vi "MAIN only-save-v3.vi"(0 "VISA resource name":refnum<visa-resource-name>="COM1", 1 "baud rate":u32=9600, 3 "bytes to read":u32=1000, 4 "data bits":u16=8 min=5 max=8 step=1, 5 "parity":u16(ring) items=["None", "Odd", "Even", "Mark", "Space"], 7 "stop bits":u16(ring)=10 items=["1.0"=10, "1.5"=15, "2.0"=20], 9 "XON Character":u8=17 format="%.0x", 13 "string to write":string="*IDN?", 14 "XOFF Character":u8=19 format="%.0x", 15 "timeout (ms)":u32=10000, 17 "write":bool=TRUE, 21 "End read on termination character?":bool=TRUE, 24 "termination char\n(0xA = '\\n' = LF)":u8=10 format="%.0x", 25 "Input\nbuffer size":u32=4096, 26 "read":bool=TRUE) -> (20 "read string":string)   [LabVIEW 2012]
doc: "The Advanced Serial Read and Write example performs a Serial Port Read, a Serial Port Write, or a combination of these actions while setting some advanced serial features like buffer size, termination characters, and XON/XOFF flow control. The user selects the actions (read or write) on the front panel. If both are selected, the VI will write the data first, read the data and then close the VISA session that is opened to the port. \n\nThe parameters set for the serial port must match the parameters of the connected instrument or device. In this example, the bytes to read parameter specifies the number of bytes that the serial port reads. If there were more bytes at the port than the number specified in bytes to read, those bytes would not be read. Also, if you specify to read more bytes than the number of bytes actually read, you might receive a timeout error message.\n\nINSTRUCTIONS:\n1) Select the serial resource and configuration parameters (baud rate, data bits, parity, stop bits, flow control).\n2) Termination character can be enabled and set. Also, set the required input buffer size prior to running the example.\n3) Select the operations to be performed. \n4) Connect the serial port to your device. If no device is available, perform a loopback test by doing one of the following. Short pins 2 and 3 on a RS-232 cable or short pin 4 to pin 8 and pin 5 to pin 9 on a RS-485/422 cable. \n5) Run the VI to see the data read. (The \"read string\" will match the \"string to write\" if a loopback test was performed.)\n\nThis example exposes several advanced features that you may need for your application. Not all applications need all the features shown in this example. The input buffer size is likely an important setting that you want to control in your application. This example expands upon the flow control option for XON and XOFF, allowing the user to choose those control characters. The timeout parameter has been brought to the front panel so a user can specify the time period the VISA Read will wait for the number of bytes to read before timing out. Also, the user has several controls for the termination character, which is discussed later.\n\nNote that you can press the write and read buttons and change the bytes to read parameters on the fly, while the example is running. However, you must stop the example to change the other configuration parameters after the example has started running, and then run again.\n\nSet the I/O buffer size slightly higher the amount of data you expect to receive. This is very important for applications that don't use flow control, as you may lose characters if the receive buffer overflows.\n\nSetting the timeout period ensures that the operation returns with a timeout error if the operation cannot be performed in the specified time period. \n\nSome devices require a termination character in order to identify the end of command strings. Some devices send a termination character to signify the end of data to be read. \n\nThis example shows how you can end the Read operation once a termination character is detected in the buffer and/or append a termination character at the end of the Write data. To enable the Read to end on a termination character, use the VISA Configure Serial Port or use the VISA Properties Serial End Mode for Reads, Termination Character Enable, and Termination Character. To end the Write with a termination character, use the VISA Properties Serial End Mode for Writes, the Send End Enable, and Termination Character. In this example, the same termination character is used for both the Read and the Write. You can specify two different characters for your application, if desired.\n\nYour application may require specific characters for the XON/XOFF Flow Control. You can specify these characters with the VISA Properties Flow Control XOFF Character and Flow Control XON Character. Note that if the standard XON and XOFF characters are used, then decimal 17 and 19 are unavailable for data values. Remember that using flow control and setting an adequate buffer size allow you to prevent buffer overflows."
uses:
  <vilib>/Instr/_visa.llb/VISA Configure Serial Port (Instr).vi
panel:
  out "actual bytes read":u32
  in  "stop":bool
  in  "flow control":u16(ring) items=["None"=0, "XON/XOFF"=1, "RTS/CTS"=2, "DTR/DSR"=4]
  in  "End write with termination character?":bool=TRUE
  # "On Windows/Linux, consider using the Instrument Driver Finder (Help>>Find Instrument Drivers) to search for an instrument driver for your instrument."
  # "Select the serial resource and the operations to be performed.  If all are selected, the VI will write the data first, read data and then close the VISA session that is opened to the port.  This VI will wait until the specified number of bytes is received at the port, until the timeout period is met, or until a termination character is received.  The default termination character in this example is the Line Feed ( ASCII 0xA, '\\n' ).  Also, set the required input buffer size prior to running the example.\nNote: The example loops until the STOP button is pressed."
  # "For additional information select File >> VI Properties >> Documentation"
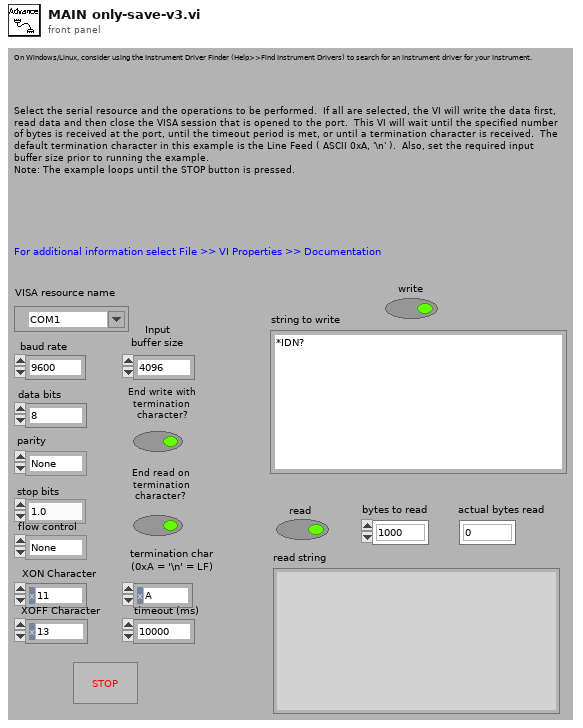
[diagram p1: front panel]
types:
  T1 = enum16{"open", "replace", "create", "open or create", "replace or create", "replace or create with confirmation"}
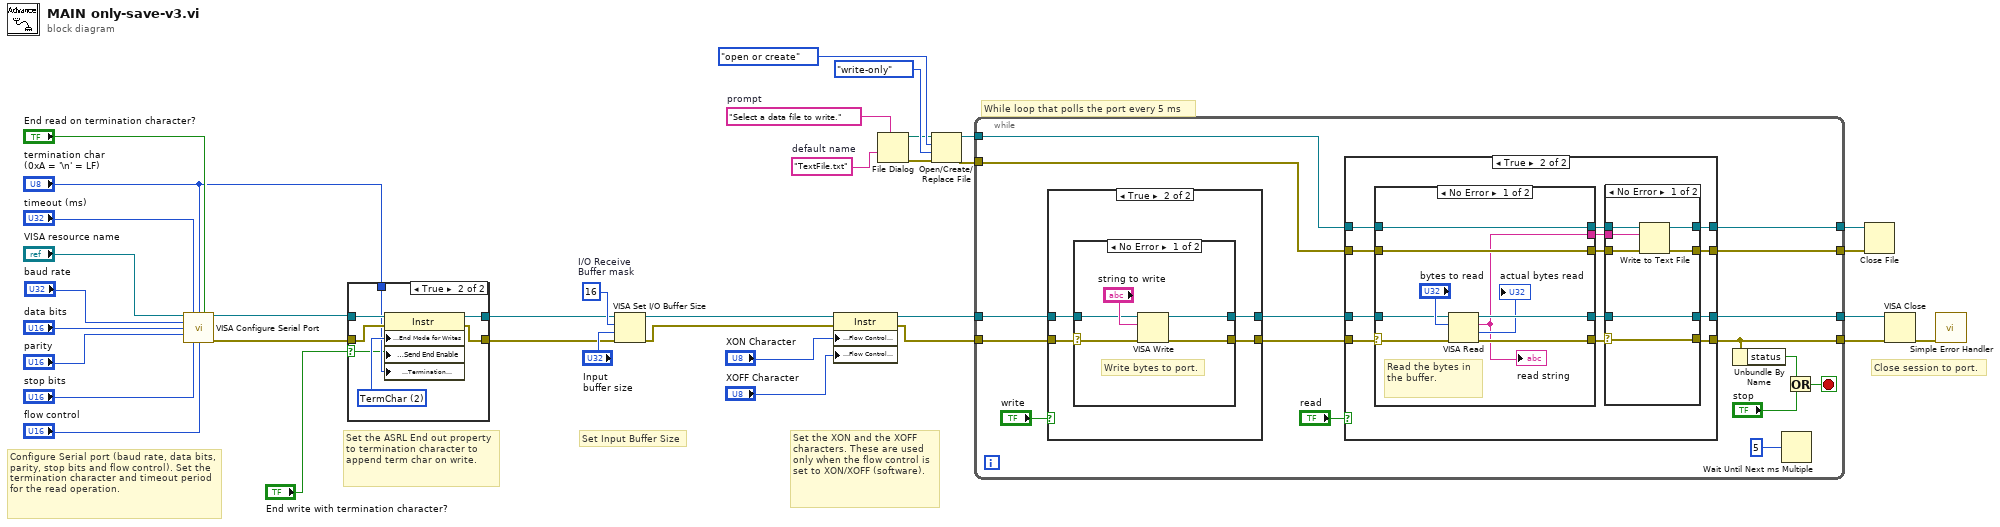
[diagram p0: block diagram]
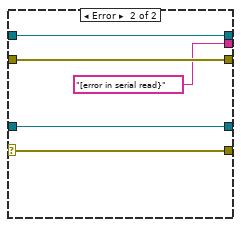
[diagram p7: hidden frame]
diagram:
  w6 = "TextFile.txt"  # default name
  w7 = "Select a data file to write."  # prompt
  w28 = u16 16  # I/O Receive Buffer mask
  # "While loop that polls the port every 5 ms"
  # "Set the XON and the XOFF characters. These are used only when the flow control is set to XON/XOFF (software)."
  # "Configure Serial port (baud rate, data bits, parity, stop bits and flow control). Set the termination character and timeout period for the read operation."
  # "Set Input Buffer Size"
  # "Set the ASRL End out property to termination character to append term char on write."
  # "Close session to port."
  n1 = call-poly "VISA Configure Serial Port"("VISA resource name"="VISA resource name", "timeout (10sec)"="timeout (ms)", "termination char\n(0xA = '\\n' = LF)"="termination char\n(0xA = '\\n' = LF)", "Enable Termination\nChar (T)"="End read on termination character?", "baud rate (9600)"="baud rate", "data bits (8)"="data bits", "parity (0:none)"="parity", "stop bits (10: 1 bit)"="stop bits", "flow control (0:none)"="flow control") -> ("VISA resource name out"=w14:refnum<visa-resource-name>, "error out"=w17:errorcluster)  [unwired: 1 in, 4 out]
  n2 = case shown="True" "End write with termination character?" {
    selector: "End write with termination character?" -> [_ w38]
    tunnel: w14 -> [w36 w44]
    tunnel: w17 -> [w37 w43]
    tunnel: [w36 w42] -> w15
    tunnel: [w37 w41] -> w16
    tunnel: "termination char\n(0xA = '\\n' = LF)" -> [_ w39]
    frame False {
    }
    frame True {
      w40 = u16 2 items=["None", "LastBit", "TermChar", "Break"] ("Serial Settings:Serial End Mode for Writes")
      n3 = property class="Instr"(reference=w44, error in=w43, "Serial Settings:End Mode for Writes"=w40, "Message Based Settings:Send End Enable"=w38, "Message Based Settings:Termination Character"=w39) -> (reference out=w42:refnum<visa-resource-name>, error out=w41:errorcluster)
    }
  }
  n4 = VISA Set I/O Buffer Size(VISA resource name=w15, mask (16)=w28, size (4096)="Input\nbuffer size", error in (no error)=w16) -> (VISA resource name out=w23:refnum<visa-resource-name>, error out=w22:errorcluster)
  n5 = property class="Instr"(reference=w23, error in=w22, "Serial Settings:Flow Control XON Character"="XON Character", "Serial Settings:Flow Control XOFF Character"="XOFF Character") -> (reference out=w13:refnum<visa-resource-name>, error out=w19:errorcluster)
  n6 = File Dialog(7:w7, 9:w6) -> (0:w8:errorcluster, 3:w5:path)  [unwired: 1 in, 6 out]
  n7 = Open/Create/Replace File(file path (use dialog)=w5, error in=w8, operation (0:open)=T1."open or create", access (0:read/write)=enum16{"read/write", "read-only", "write-only"}."write-only") -> (refnum out=w1:refnum<file>, error out=w2:errorcluster)  [unwired: 3 out]
  n8 = while {
    tunnel: w19 -> [w53]
    tunnel: w13 -> [w54]
    tunnel: [w52] -> w12
    tunnel: [w51] -> w11
    tunnel: [w48] -> w4
    tunnel: [w47] -> w3
    tunnel: w2 -> [w45]
    tunnel: w1 -> [w46]
    stop <- w50 stop-if-true
    n9 = case shown="True" "write" {
      tunnel: [w62 w66] -> w57
      tunnel: [w61 w65] -> w56
      tunnel: w54 -> [w62 w64]
      tunnel: w53 -> [w61 w63]
      frame False {
      }
      frame True {
        n10 = case shown="No Error" w63 {
          selector: w63 -> [w67 w73]
          tunnel: [w71 w72] -> w66
          tunnel: [w70 w73] -> w65
          tunnel: w64 -> [w68 w72]
          frame No Error {
            # "Write bytes to port."
            n11 = VISA Write(VISA resource name=w68, write buffer="string to write", error in (no error)=w67) -> (VISA resource name out=w71:refnum<visa-resource-name>, error out=w70:errorcluster)  [unwired: 1 out]
          }
          frame Error {
          }
        }
      }
    }
    n12 = case shown="True" "read" {
      tunnel: w56 -> [w76 w90]
      tunnel: w57 -> [w77 w89]
      tunnel: [w76 w79] -> w51
      tunnel: [w77 w81] -> w52
      tunnel: [w74 w83] -> w48
      tunnel: [w75 w85] -> w47
      tunnel: w46 -> [w75 w88]
      tunnel: w45 -> [w74 w87]
      frame False {
      }
      frame True {
        n13 = case "Read bytes from port." shown="No Error" w90 {
          selector: w90 -> [w106 w114]
          tunnel: [w109 w114] -> w80
          tunnel: [w110 w115] -> w82
          tunnel: w89 -> [w107 w115]
          tunnel: [w104 w112] -> w84
          tunnel: [w102 w113] -> w86
          tunnel: w88 -> [w102 w113]
          tunnel: w87 -> [w104 w112]
          tunnel: [w103 "[error in serial read}" ("read buffer")] -> w78
          frame No Error {
            # "Read the bytes in the buffer."
            n14 = VISA Read(VISA resource name=w107, byte count="bytes to read", error in (no error)=w106) -> (VISA resource name out=w110:refnum<visa-resource-name>, read buffer=w103:string, return count=→"actual bytes read":u32, error out=w109:errorcluster)
            "read string" <- w103
          }
          frame Error {
            # "Error occurred \nreading Bytes at \nSerial Port"
          }
        }
        n15 = case "Read bytes from port." shown="No Error" w80 {
          selector: w80 -> [w97 w98]
          tunnel: [w97 w98] -> w79
          tunnel: w86 -> [w92 w101]
          tunnel: [w91 w101] -> w85
          tunnel: w84 -> [w95 w100]
          tunnel: [w94 w100] -> w83
          tunnel: w82 -> [w96 w99]
          tunnel: [w96 w99] -> w81
          tunnel: w78 -> [w93 _]
          frame No Error {
            n16 = Write to Text File(file (use dialog)=w92, text=w93, error in=w95) -> (refnum out=w91:refnum<file>, error out=w94:errorcluster)  [unwired: 1 in, 1 out]
          }
          frame Error {
            # "Error occurred \nreading Bytes at \nSerial Port"
          }
        }
      }
    }
    n17 = Unbundle By Name(w51) -> ("status"=w58:bool)
    n18 = Wait Until Next ms Multiple(millisecond multiple=u32 5) -> ()  [unwired: 1 out]
    n19 = Or(x=w58, y="stop") -> (x .or. y?=w50:bool)
  }
  n20 = Close File(refnum=w3, error in=w4) -> ()  [unwired: 2 out]
  n21 = VISA Close(VISA resource name=w12, error in (no error)=w11) -> (error out=w33:errorcluster)
  n22 = call <vilib>:"Simple Error Handler.vi"("error in (no error)"=w33) -> ()  [unwired: 1 in, 8 out]
